vi "Handle Error.vi"(8 "error in (no error)":errorcluster, 11 "BuildWorker in":refnum<class "BuildWorker.lvclass">) -> (0 "error out":errorcluster, 2 "stop actor?":bool=TRUE, 3 "BuildWorker out":refnum<class "BuildWorker.lvclass">)   [LabVIEW 2017, in "BuildWorker.lvlib" / "BuildWorker.lvclass"]
doc: "(<B>Filename</B>: Actor Framework.lvlib:Actor.lvclass:Handle Error.vi)\n\nDefines how the actor handles an error that occurred while processing a message. By default, this method does nothing except stop the actor."
uses:
  BuildWorker.lvclass
  <vilib>/Utility/error.llb/DialogType.ctl
  BuildWorker.lvclass/BuildWorker.ctl
  Framework/Actor wUI/Actor wUI.lvclass
  BuildWorker Messages/Send Worker Status Update Msg/Send Worker Status Update Msg.lvclass
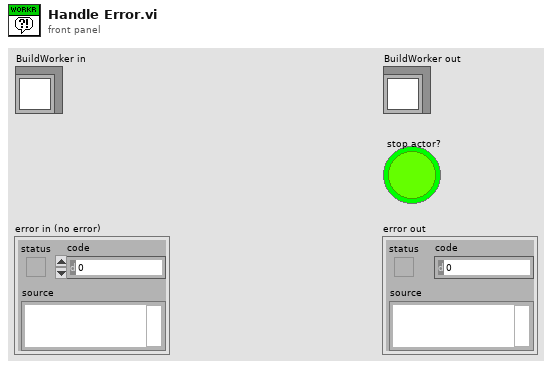
[diagram p1: front panel]
types:
  T1 = typedef "DialogType.ctl" = u16
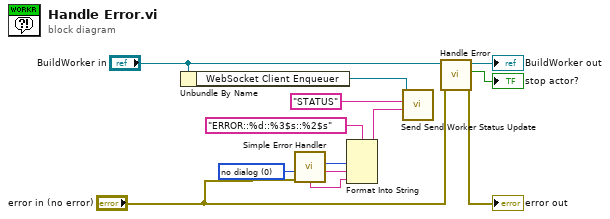
[diagram p0: block diagram]
diagram:
  w8 = T1 0 items=["no dialog", "OK message", "continue or stop message", "OK message + warnings", "continue/stop + warnings"] ("type of dialog (OK msg:1)")
  n1 = Unbundle By Name("BuildWorker in") -> ("WebSocket Client Enqueuer"=w9:refnum<class "Message Enqueuer.lvclass">)
  n2 = call <vilib>:"Simple Error Handler.vi"("type of dialog (OK msg:1)"=w8, "error in (no error)"="error in (no error)") -> ("code out"=w7:i32, "source out"=w6:string, "message"=w5:string)  [unwired: 3 in, 2 out]
  n3 = Format Into String(format string="ERROR::%d::%3$s::%2$s", w7, w6, w5) -> (resulting string=w3:string)  [unwired: 2 in, 1 out]
  n4 = call "Send Send Worker Status Update.vi"("Status"=w3, "Operation"="STATUS", "Message Enqueuer in"=w9) -> ()  [unwired: 7 in, 2 out]
  n5 = call-parent "Handle Error.vi"("error in (no error)"="error in (no error)", "Actor in"="BuildWorker in") -> ("error out"=→"error out":errorcluster, "stop actor?"=→"stop actor?":bool, "Actor out"=→"BuildWorker out":refnum<class "BuildWorker.lvclass">)  [unwired: 7 in]
